vi "Keithley 2002 Arm2 Config.vi"(2 "async output (line 1:0)":u16(ring) items=["line 1", "line 2", "line 3", "line 4", "line 5", "line 6"], 3 "async input (line 2:1)":u16(ring)=1 items=["line 1", "line 2", "line 3", "line 4", "line 5", "line 6"], 4 "timer value (secs)":dbl=1.0 min=0.001 max=999999.999 format="%.3f", 5 "count value":dbl=1.0 min=1.0 max=99999.0 step=1.0, 6 "source (imm:1)":u16(ring)=1 items=["hold", "immediate", "timer", "manual", "bus", "trigger link", "external"], 7 "count (set:0)":u16(ring) items=["set  value", "infinite", "min", "max"], 8 "error in":T1, 9 "delay (secs)":dbl min=0.0 max=999999.999 format="%.3f", 10 "direction":bool, 11 "GPIB address":string="16") -> (0 "error out":T1)   [LabVIEW 2020]
doc: "This VI is used to configure the settings for the Scan Layer (Arm2) of the trigger model. The model consists of 3 layers, the Arm Layer, the Scan Layer (Arm2), and the Measure Layer (Trigger).\n\nIn general, the instrument requires a scan event to allow operation to proceed to the next layer (Trigger)."
panel:
  # "source\nacceptor"
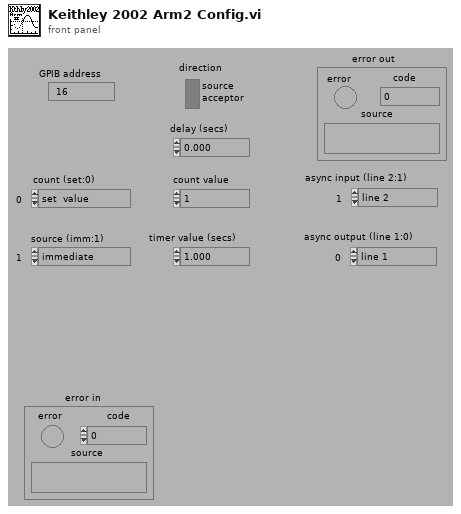
[diagram p1: front panel]
types:
  T1 = cluster{"error":bool, "code":i32, "source":string}
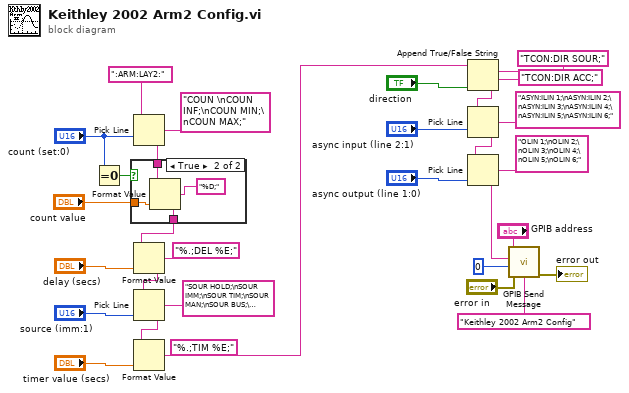
[diagram p0: block diagram]
diagram:
  n1 = Equal To 0?(x="count (set:0)") -> (x = 0?=w22:bool)
  n2 = Pick Line(string ("")=":ARM:LAY2:", multi-line string="COUN \nCOUN INF;\nCOUN MIN;\nCOUN MAX;", line index="count (set:0)") -> (output string=w23:string)
  n3 = case shown="True" w22 {
    tunnel: "count value" -> [_ w36]
    tunnel: w23 -> [w32 w35]
    tunnel: [w32 w33] -> w8
    frame False {
    }
    frame True {
      n4 = Format Value(string ("")=w35, format string="%D;", value (0)=w36) -> (output string=w33:string)
    }
  }
  n5 = Format Value(string ("")=w8, format string="%.;DEL %E;", value (0)="delay (secs)") -> (output string=w7:string)
  n6 = Pick Line(string ("")=w7, multi-line string="SOUR HOLD;\nSOUR IMM;\nSOUR TIM;\nSOUR MAN;\nSOUR BUS;\nSOUR TLIN;\nSOUR EXT;", line index="source (imm:1)") -> (output string=w4:string)
  n7 = Format Value(string ("")=w4, format string="%.;TIM %E;", value (0)="timer value (secs)") -> (output string=w2:string)
  n8 = Append True/False String(1:"direction", 2:"TCON:DIR ACC;", 3:"TCON:DIR SOUR;", 4:w2) -> (0:w11:string)
  n9 = Pick Line(string ("")=w11, multi-line string="ASYN:ILIN 1;\nASYN:ILIN 2;\nASYN:ILIN 3;\nASYN:ILIN 4;\nASYN:ILIN 5;\nASYN:ILIN 6;", line index="async input (line 2:1)") -> (output string=w13:string)
  n10 = Pick Line(string ("")=w13, multi-line string="OLIN 1;\nOLIN 2;\nOLIN 3;\nOLIN 4;\nOLIN 5;\nOLIN 6;", line index="async output (line 1:0)") -> (output string=w3:string)
  n11 = call "GPIB Send Message.vi"("address string"="GPIB address", "write buffer"=w3, "source"="Keithley 2002 Arm2 Config", "write mode (set END:0)"=0, "error in"="error in") -> ("error out"=→"error out":T1)  [unwired: 2 in, 2 out]
